vi "DefaultFromIni.vi"(8 "error in (no error)":errorcluster, 11 "SyncPlugin":refnum<class "NiPxi6683H.lvclass">) -> (0 "error out":errorcluster, 3 "SyncPlugin":refnum<class "NiPxi6683H.lvclass">)   [LabVIEW 2014, in "SyncPlugins.lvlib" / "NiPxi6683H.lvclass"]
uses:
  NiPxi6683H.lvclass
  PXI_MultiTrig/Typedefs/clTrigger.ctl
  PXI_MultiTrig/Typedefs/clClocks.ctl
  PXI_MultiTrig/Typedefs/TimeRefType.ctl
  <userlib>/NIST/BaseClasses/BasePlugin_class/BasePlugin.lvclass/BasePlugin.ctl
  NiPxi6683H.lvclass/NiPxi6683H.ctl
  <userlib>/NIST/BaseClasses/BasePlugin_class/Accessors/Read PluginIniFilePath.vi
  Accessors/Write Triggers.vi
  Accessors/Write Clocks.vi
  Accessors/Write TimeRefType.vi
  NiPxi6682/NiPxi6682.lvclass
  <vilib>/Utility/config.llb/NI_LVConfig.lvlib
  PXI_MultiTrig/PXI_MultiTrig.lvclass
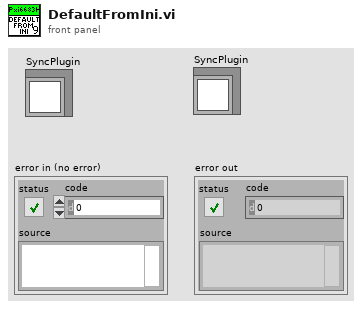
[diagram p1: front panel]
types:
  T1 = typedef "SyncPlugins.lvlib/PXI_MultiTrig.lvclass/TimeRefType.ctl" = enum16{"1588", "Free Running", "GPS", "IRIG", "PPS"}
  T2 = typedef "SyncPlugins.lvlib/PXI_MultiTrig.lvclass/clClocks.ctl" = cluster{"Name":string, "RefClk":string, "ClkTerminal":string, "Frequency":dbl, "DutyCycle":dbl, "ClkType":string, "Initiated":bool, "TrigTime":bool}
  T3 = typedef "SyncPlugins.lvlib/PXI_MultiTrig.lvclass/clTrigger.ctl" = cluster{"Name":string, "DestTerm":string, "SrcTerm":string, "SyncClk":string, "Edge":i32, "Invert?":i32, "Initiated":bool, "Type":string, "TrigTime":bool}
  T4 = typedef "NI_LVConfig.lvlib/Config Data RefNum.ctl" = refnum<k1>
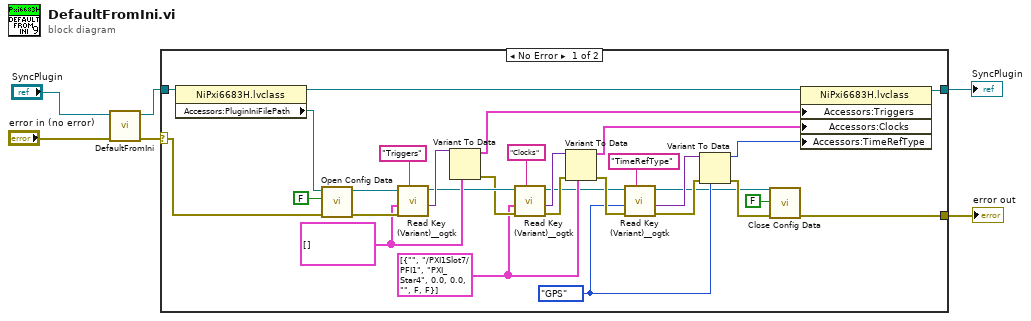
[diagram p0: block diagram]
diagram:
  n1 = call-parent "DefaultFromIni.vi"("error in (no error)"="error in (no error)", "SyncPlugin"="SyncPlugin") -> ("error out"=w4:errorcluster, "SyncPlugin"=w3:refnum<class "NiPxi6683H.lvclass">)  [unwired: 8 in]
  n2 = case shown="No Error" w4 {
    selector: w4 -> [w34 w37]
    tunnel: w3 -> [w36 w38]
    tunnel: [w16 w37] -> w1
    tunnel: [w27 w38] -> w2
    frame No Error {
      w11 = TimeRefType."GPS" ("TimeRefType")
      w19 = T2[] [{"Name"="", "RefClk"="/PXI1Slot7/PFI1", "ClkTerminal"="PXI_Star4", "Frequency"=0.0, "DutyCycle"=0.0, "ClkType"="", "Initiated"=FALSE, "TrigTime"=FALSE}]
      w25 = T3[] []
      n3 = property class="NiPxi6683H.lvclass"(reference=w36) -> (reference out=w31:refnum<class "NiPxi6683H.lvclass">, "Accessors:PluginIniFilePath"=w35:path)  [unwired: 1 in, 1 out]
      n4 = call <vilib>:"Open Config Data.vi"("error in (no error)"=w34, "create file if necessary (T)"=FALSE, "configuration file path"=w35) -> ("error out"=w32:errorcluster, "refnum"=w29:T4)  [unwired: 6 in, 1 out]
      n5 = call <userlib>:"Read Key (Variant)__ogtk.vi"("section"="Triggers", "error in (no error)"=w32, "type"=w25, "refnum"=w29) -> ("key-value"=w26:variant, "refnum out"=w23:T4)  [unwired: 4 in, 2 out]
      n6 = Variant To Data(type=w25, Variant=w26) -> (data=w24:T3[], error out=w21:errorcluster)  [unwired: 1 in]
      n7 = call <userlib>:"Read Key (Variant)__ogtk.vi"("section"="Clocks", "error in (no error)"=w21, "type"=w19, "refnum"=w23) -> ("error out"=w20:errorcluster, "key-value"=w17:variant, "refnum out"=w7:T4)  [unwired: 4 in, 1 out]
      n8 = Variant To Data(error in=w20, type=w19, Variant=w17) -> (data=w18:T2[], error out=w15:errorcluster)
      n9 = call <userlib>:"Read Key (Variant)__ogtk.vi"("section"="TimeRefType" ("key (optional)"), "error in (no error)"=w15, "type"=w11, "refnum"=w7) -> ("error out"=w12:errorcluster, "key-value"=w13:variant, "refnum out"=w8:T4)  [unwired: 4 in, 1 out]
      n10 = Variant To Data(error in=w12, type=w11, Variant=w13) -> (data=w9:T1, error out=w10:errorcluster)
      n11 = call <vilib>:"Close Config Data.vi"("error in (no error)"=w10, "write file if changed (T)"=FALSE ("create file if necessary (T)"), "refnum"=w8) -> ("error out"=w16:errorcluster)  [unwired: 7 in, 1 out]
      n12 = property class="NiPxi6683H.lvclass"(reference=w31, "Accessors:Triggers"=w24, "Accessors:Clocks"=w18, "Accessors:TimeRefType"=w9) -> (reference out=w27:refnum<class "NiPxi6683H.lvclass">)  [unwired: 1 in, 1 out]
    }
    frame Error {
    }
  }
  "SyncPlugin" <- w2
  "error out" <- w1
